vi "Do.vi"(8 "error in (no error)":errorcluster, 10 "Actor in":refnum<class "Actor.lvclass">, 11 "Ack Completion Long Exec Meth Msg in":refnum<class "Ack Completion Long Exec Meth Msg.lvclass">) -> (0 "error out":errorcluster, 2 "Actor out":refnum<class "Actor.lvclass">)   [LabVIEW 2021, in "Async Methods Actor Example.lvlib" / "Ack Completion Long Exec Meth Msg.lvclass"]
doc: "(<B>Filename</B>: Actor Framework.lvlib:Message.lvclass:Do.vi)\n\nDefines what a message does when it is received by an actor. Generally, a message instructs an actor to invoke one of its methods. By default, this method does nothing. A child class must override it to define behavior. Create a child class by using the Actor Framework Message Maker dialog box."
uses:
  Ack Completion Long Exec Meth Msg.lvclass
  C:/Projects/Async Methods Actor/Async Methods Actor/Async Methods Actor Messages/Completion Notification Msg/Completion Notification Msg.lvclass
  <vilib>/ActorFramework/Actor/Actor.lvclass
  Async Methods Actor Example/Async Methods Actor Example.lvclass
  C:/Program Files/National Instruments/LabVIEW 2021/vi.lib/ActorFramework/Actor/Actor.lvclass
  Async Methods Actor/Async Methods Actor Messages/Completion Notification Msg/Completion Notification Data.ctl
  Async Methods Actor/Async Methods Actor Messages/Async Message/Async Message.lvclass
  Async Methods Actor/Async Methods Actor Messages/Completion Notification Msg/Completion Notification Msg.lvclass/Completion Notification Msg.ctl
  Async Methods Actor/Async Methods Actor Messages/Completion Notification Msg/Read Async Message.vi
  Async Methods Actor/Async Methods Actor Messages/Completion Notification Msg/w.vi
  Async Methods Actor/Async Methods Actor Messages/Completion Notification Msg/Completion Notification Msg.lvclass
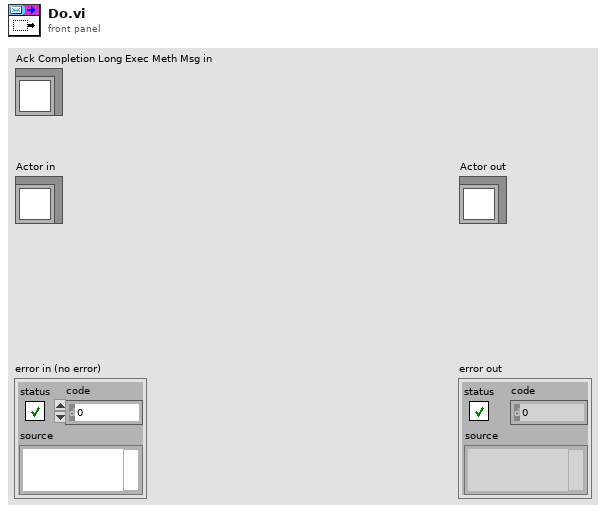
[diagram p1: front panel]
types:
  T1 = typedef "Async Methods Actor.lvlib/Completion Notification Msg.lvclass/Completion Notification Data.ctl" = cluster{"Async Message":refnum<class "Async Message.lvclass">, "Current Execution Count":u32}
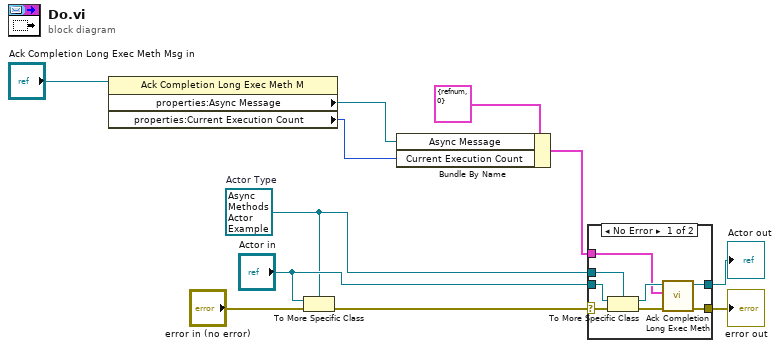
[diagram p0: block diagram]
diagram:
  w6 = refnum<class "Async Methods Actor Example.lvclass"> refnum  # Actor Type
  n1 = property class="Ack Completion Long Exec Meth M"(reference="Ack Completion Long Exec Meth Msg in") -> ("properties:Async Message"=w2:refnum<class "Async Message.lvclass">, "properties:Current Execution Count"=w1:u32)  [unwired: 1 in, 2 out]
  n2 = To More Specific Class(target class=w6, reference="Actor in", error in="error in (no error)") -> (error out=w10:errorcluster)  [unwired: 1 out]
  n3 = Bundle By Name(cluster=T1 {"Async Message"=refnum, "Current Execution Count"=0} ("Completion Ack Data"), "Async Message"=w2, "Current Execution Count"=w1) -> (w3:T1)
  n4 = case shown="No Error" w10 {
    selector: w10 -> [w19 w21]
    tunnel: [w14 w21] -> w9
    tunnel: [w13 w20] -> w8
    tunnel: "Actor in" -> [w18 w20]
    tunnel: w6 -> [w17 _]
    tunnel: w3 -> [w12 _]
    frame No Error {
      n5 = To More Specific Class ("Actor Cast")(target class=w17, reference=w18, error in=w19) -> (specific class reference=w16:refnum<class "Async Methods Actor Example.lvclass">, error out=w15:errorcluster)
      n6 = call "Ack Completion Long Exec Meth.vi"("error in (no error)"=w15, "Completion Ack Data"=w12, "Async Methods Actor Example in"=w16) -> ("error out"=w14:errorcluster, "Async Methods Actor Example out"=w13:refnum<class "Async Methods Actor Example.lvclass">)  [unwired: 7 in]
    }
    frame Error {
    }
  }
  "error out" <- w9
  "Actor out" <- w8
